vi "Pre Launch Init.vi"(11 "Range Controller Actor in":refnum<class "Range Controller Actor.lvclass">) -> (0 "error out":errorcluster, 3 "Range Controller Actor out":refnum<class "Range Controller Actor.lvclass">)   [LabVIEW 2018, in "Range Controller.lvlib" / "Range Controller Actor.lvclass"]
doc: "Sends a high priority message to it's self to notify the monitor that it's spawned. If it's in the runtime environment, this message is never sent, meaning the monitor will never spawn\n\nCopyright: MGI\nAuthored by: Derek Trepanier"
uses:
  Range Controller Actor.lvclass
  Range Controller Actor.lvclass/Range Controller Actor.ctl
  Actor Monitor/Actor/Monitored Actor.lvclass
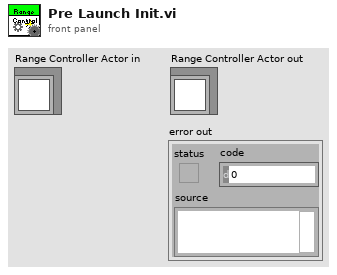
[diagram p1: front panel]
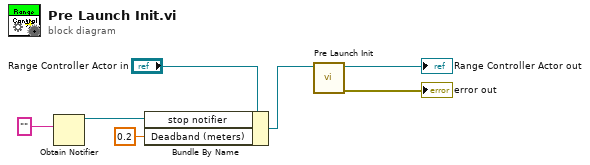
[diagram p0: block diagram]
diagram:
  n1 = Obtain Notifier(notification data type="" ("name (unnamed)")) -> (notifier out=w3:refnum<notifier>)  [unwired: 3 in, 2 out]
  n2 = Bundle By Name(cluster="Range Controller Actor in", "stop notifier"=w3, "Deadband (meters)"=0.2) -> (w4:refnum<class "Range Controller Actor.lvclass">)
  n3 = call-parent "Pre Launch Init.vi"("Monitored Actor in"=w4) -> ("error out"=→"error out":errorcluster, "Monitored Actor out"=→"Range Controller Actor out":refnum<class "Range Controller Actor.lvclass">)  [unwired: 9 in]
